vi "Objective scan control.vi"() -> ()   [LabVIEW 2012]
panel:
  in  "Stop":dbl
  in  "Pause Button":bool
  in  "Scan":bool
  in  "Start":dbl
  in  "Stop Button":bool
  in  "Step size":dbl=1.0
  in  "Previous Button":bool
  in  "Next Button":bool
  in  "Move Absolute":bool=TRUE
  out "Position":dbl[](array[numeric])=[-1.0] format="%.6f"
  in  "Absolute":dbl=50.0
  in  "RS232 settings":cluster{"Portnumber":i32, "Baudrate":u16}={"Portnumber"=6, "Baudrate"=5} {"Portnumber" items=["COM1", "COM2", "COM3", "COM4", "COM5", "COM6", "COM7", "COM8", "COM9", "COM10", "COM11", "COM12", "COM13", "COM14", "COM15", "COM16", "COM17", "COM18", "COM19", "COM20", "COM21", "COM22", "COM23", "COM24", "COM25", "COM26", "COM27", "COM28", "COM29", "COM30"]; "Baudrate" items=["9600", "14400", "19200", "38400", "57600", "115200"]}
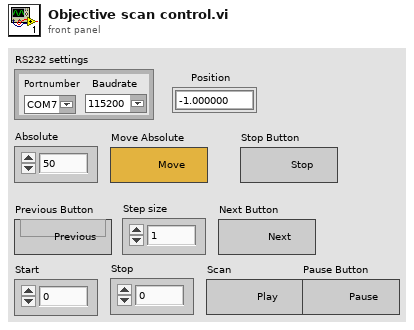
[diagram p1: front panel]
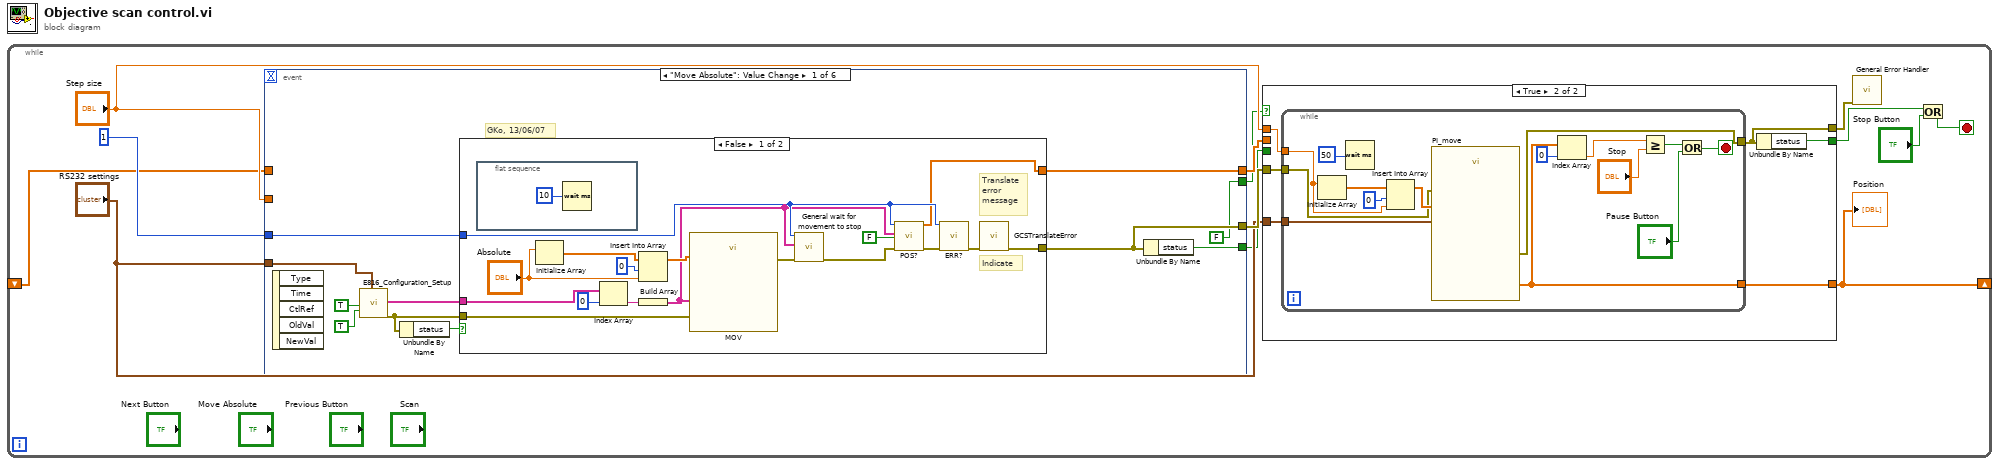
[diagram p0: block diagram]
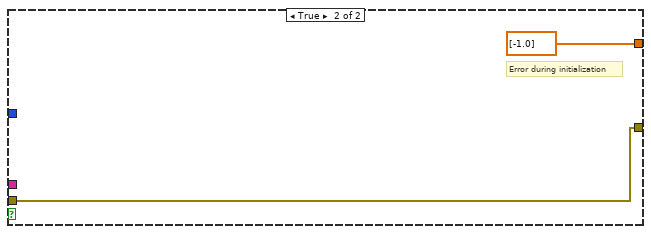
[diagram p3: hidden frame]
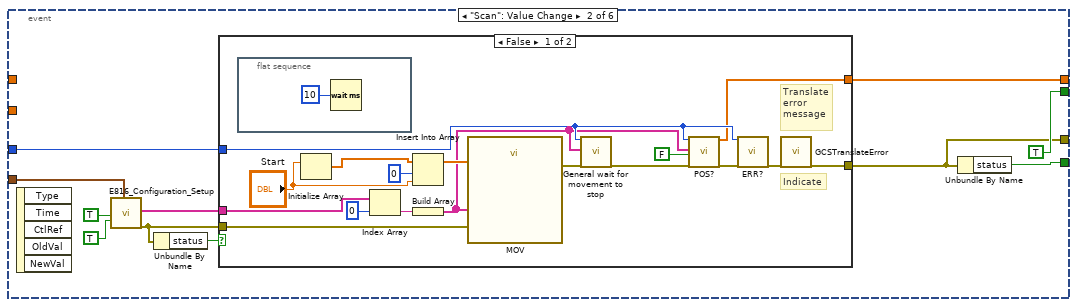
[diagram p4: hidden frame]
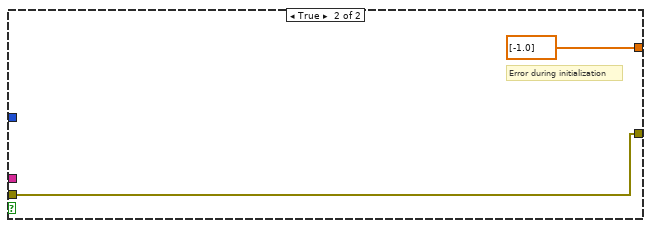
[diagram p5: hidden frame]
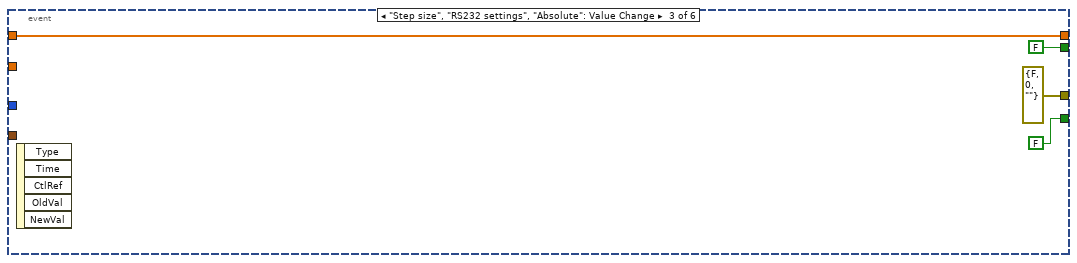
[diagram p6: hidden frame]
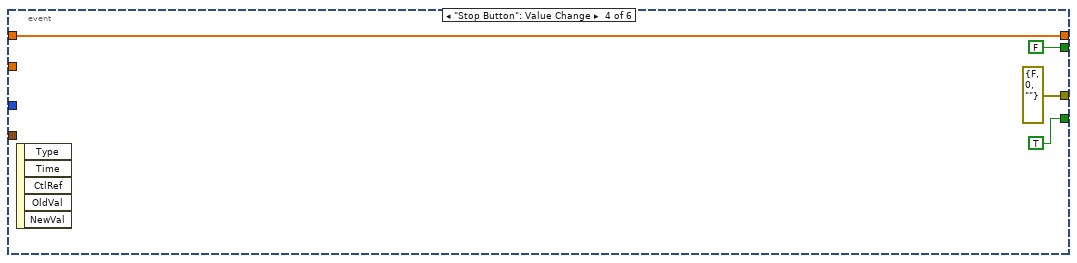
[diagram p7: hidden frame]
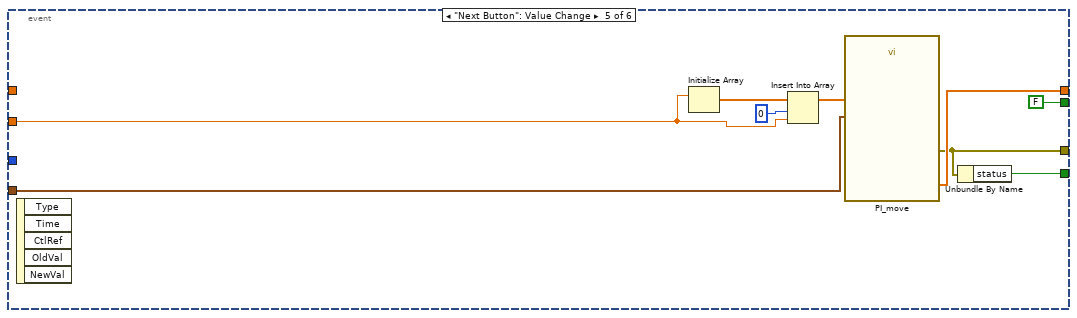
[diagram p8: hidden frame]
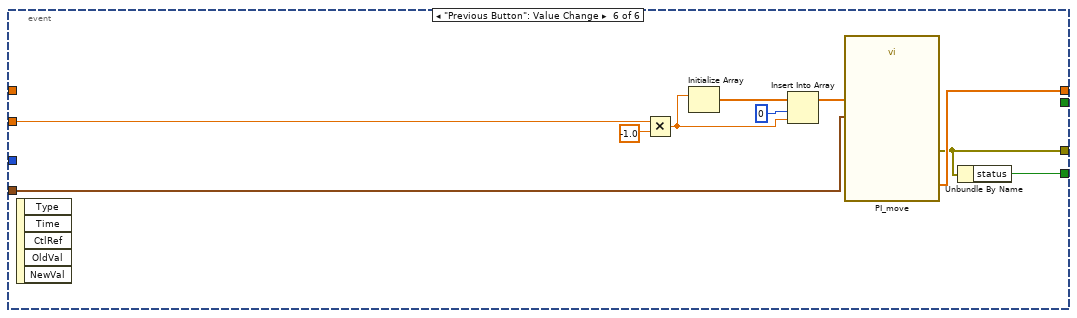
[diagram p9: hidden frame]
diagram:
  n1 = while {
    shift-right: [w2] -> _
    shift-left: _ -> [w1]
    stop <- w11 stop-if-true
    n2 = event shown="[0] \"Move Absolute\": Value Change" {
      selector: _ -> [_ _ _ _ _ _]
      dyn-events: _ -> [_ _ _ _ _ _]
      timeout: _ -> [_ _ _ _ _ _]
      tunnel: 1 ("System no.") -> [w48 w76 _ _ _ _]
      tunnel: [w40 w69 errorcluster {"status"=FALSE, "code"=0, "source"=""} ("error out") errorcluster {"status"=FALSE, "code"=0, "source"=""} ("error out") w110 w120] -> w10
      tunnel: "RS232 settings" -> [w46 w73 _ _ w113 w123]
      tunnel: [w42 w72 w100 w104 w112 w121] -> w7
      tunnel: "Step size" -> [_ _ _ _ w111 w122]
      tunnel: [w39 w70 FALSE ("status") TRUE ("status") w109 w119] -> w5
      tunnel: [FALSE TRUE FALSE FALSE FALSE _] -> w6
      tunnel: w1 -> [_ _ w100 w104 _ _]
      event "Move Absolute": Value Change {
        # "GKo, 13/06/07"
        n3 = event-data() -> ()  [unwired: 1 in, 5 out]
        n4 = call "E816_Configuration_Setup.vi"("All axes?"=TRUE, "Change servo \nstatus to ON?"=TRUE ("Change servo \nstatus to ON?"), "RS232 settings"=w46) -> ("Conn. Axes"=w45:string[], "error out"=w41:errorcluster)  [unwired: 13 in, 2 out]
        n5 = Unbundle By Name(w41) -> ("status"=w47:bool)
        n6 = case shown="False" w47 {
          tunnel: [w64 w68] -> w40
          tunnel: w48 -> [w61 _]
          tunnel: w45 -> [w50 _]
          tunnel: w41 -> [w54 w68]
          tunnel: [w53 dbl[] [-1.0] ("Position")] -> w42
          frame False {
            # "Translate\nerror \nmessage"
            # "Indicate"
            n7 = flat-sequence {
              frame #0 {
                n8 = Wait (ms)(milliseconds to wait=u32 10) -> ()  [unwired: 1 out]
              }
            }
            n9 = Initialize Array("Absolute") -> (w57:dbl[])  [unwired: 1 in]
            n10 = Index Array(array=w50, index=0) -> (element=w51:string)
            n11 = Insert Into Array(array=w57, index=0, new element="Absolute") -> (w56:dbl[])
            n12 = Build Array(w51) -> (w49:string[])
            n13 = call "MOV.vi"("Axes to move"=w49, "Position values"=w56, "error in"=w54) -> ("error out"=w59:errorcluster)  [unwired: 16 in]
            n14 = call "General wait for movement to stop.vi"("System no."=w61, "Axes to wait for"=w49, "error in"=w59) -> ("error out"=w60:errorcluster)  [unwired: 15 in, 1 out]
            n15 = call "POS?.vi"("System no."=w61, "Axes to query"=w49, "All axes?"=FALSE, "error in"=w60) -> ("Position"=w53:dbl[], "error out"=w63:errorcluster)  [unwired: 14 in]
            n16 = call "ERR?.vi"("System no."=w61, "error in"=w63) -> ("error out"=w62:errorcluster)  [unwired: 16 in, 1 out]
            n17 = call "GCSTranslateError.vi"("error in"=w62) -> ("error out"=w64:errorcluster)  [unwired: 16 in, 2 out]
          }
          frame True {
            # "Error during initialization"
          }
        }
        n18 = Unbundle By Name(w40) -> ("status"=w39:bool)
      }
      event "Scan": Value Change {
        n19 = event-data() -> ()  [unwired: 1 in, 5 out]
        n20 = call "E816_Configuration_Setup.vi"("All axes?"=TRUE, "Change servo \nstatus to ON?"=TRUE ("Change servo \nstatus to ON?"), "RS232 settings"=w73) -> ("Conn. Axes"=w77:string[], "error out"=w75:errorcluster)  [unwired: 13 in, 2 out]
        n21 = Unbundle By Name(w75) -> ("status"=w74:bool)
        n22 = case shown="False" w74 {
          tunnel: [w95 w98] -> w69
          tunnel: w76 -> [w92 _]
          tunnel: w77 -> [w83 _]
          tunnel: [w86 dbl[] [-1.0] ("Position")] -> w72
          tunnel: w75 -> [w80 w98]
          frame False {
            # "Translate\nerror \nmessage"
            # "Indicate"
            n23 = flat-sequence {
              frame #0 {
                n24 = Wait (ms)(milliseconds to wait=u32 10) -> ()  [unwired: 1 out]
              }
            }
            n25 = Initialize Array("Start") -> (w88:dbl[])  [unwired: 1 in]
            n26 = Index Array(array=w83, index=0) -> (element=w84:string)
            n27 = Insert Into Array(array=w88, index=0, new element="Start") -> (w87:dbl[])
            n28 = Build Array(w84) -> (w82:string[])
            n29 = call "MOV.vi"("Axes to move"=w82, "Position values"=w87, "error in"=w80) -> ("error out"=w90:errorcluster)  [unwired: 16 in]
            n30 = call "General wait for movement to stop.vi"("System no."=w92, "Axes to wait for"=w82, "error in"=w90) -> ("error out"=w91:errorcluster)  [unwired: 15 in, 1 out]
            n31 = call "POS?.vi"("System no."=w92, "Axes to query"=w82, "All axes?"=FALSE, "error in"=w91) -> ("Position"=w86:dbl[], "error out"=w94:errorcluster)  [unwired: 14 in]
            n32 = call "ERR?.vi"("System no."=w92, "error in"=w94) -> ("error out"=w93:errorcluster)  [unwired: 16 in, 1 out]
            n33 = call "GCSTranslateError.vi"("error in"=w93) -> ("error out"=w95:errorcluster)  [unwired: 16 in, 2 out]
          }
          frame True {
            # "Error during initialization"
          }
        }
        n34 = Unbundle By Name(w69) -> ("status"=w70:bool)
      }
      event "Step size", "RS232 settings", "Absolute": Value Change {
        n35 = event-data() -> ()  [unwired: 1 in, 5 out]
      }
      event "Stop Button": Value Change {
        n36 = event-data() -> ()  [unwired: 1 in, 5 out]
      }
      event "Next Button": Value Change {
        n37 = event-data() -> ()  [unwired: 1 in, 5 out]
        n38 = Initialize Array(w111) -> (w115:dbl[])  [unwired: 1 in]
        n39 = Insert Into Array(array=w115, index=0, new element=w111) -> (w114:dbl[])
        n40 = call "PI_move.vi"("RS232 settings"=w113, "Position values"=w114) -> ("Position"=w112:dbl[], "error out"=w110:errorcluster)  [unwired: 15 in, 1 out]
        n41 = Unbundle By Name(w110) -> ("status"=w109:bool)
      }
      event "Previous Button": Value Change {
        n42 = event-data() -> ()  [unwired: 1 in, 5 out]
        n43 = Multiply(x=w122, y=-1.0) -> (x*y=w118:dbl)
        n44 = Initialize Array(w118) -> (w125:dbl[])  [unwired: 1 in]
        n45 = Insert Into Array(array=w125, index=0, new element=w118) -> (w126:dbl[])
        n46 = call "PI_move.vi"("RS232 settings"=w123, "Position values"=w126) -> ("Position"=w121:dbl[], "error out"=w120:errorcluster)  [unwired: 15 in, 1 out]
        n47 = Unbundle By Name(w120) -> ("status"=w119:bool)
      }
    }
    n48 = case shown="True" w6 {
      tunnel: w10 -> [w15 w22]
      tunnel: "RS232 settings" -> [_ w21]
      tunnel: "Step size" -> [_ w20]
      tunnel: [w16 w19] -> w2
      tunnel: w7 -> [w16 _]
      tunnel: [w15 w17] -> w3
      tunnel: [w14 w18] -> w4
      tunnel: w5 -> [w14 _]
      frame False {
      }
      frame True {
        n49 = while {
          tunnel: w22 -> [w35]
          tunnel: [w30] -> w19
          tunnel: [w27] -> w17
          tunnel: w21 -> [w26]
          tunnel: w20 -> [w23]
          stop <- w33 stop-if-true
          n50 = Initialize Array(w23) -> (w24:dbl[])  [unwired: 1 in]
          n51 = Wait (ms)(milliseconds to wait=u32 50) -> ()  [unwired: 1 out]
          n52 = Insert Into Array(array=w24, index=0, new element=w23) -> (w36:dbl[])
          n53 = call "PI_move.vi"("RS232 settings"=w26, "Position values"=w36, "error in"=w35) -> ("Position"=w30:dbl[], "error out"=w27:errorcluster)  [unwired: 14 in, 1 out]
          n54 = Index Array(array=w30, index=0) -> (element=w28:dbl)
          n55 = Greater Or Equal?(x=w28, y="Stop") -> (x >= y?=w31:bool)
          n56 = Or(x=w31, y="Pause Button") -> (x .or. y?=w33:bool)
        }
        n57 = Unbundle By Name(w17) -> ("status"=w18:bool)
      }
    }
    "Position" <- w2
    n58 = call <vilib>:"General Error Handler.vi"("error in (no error)"=w3) -> ()  [unwired: 10 in, 5 out]
    n59 = Or(x=w4, y="Stop Button") -> (x .or. y?=w11:bool)
  }
